vi "user_PW_dialog.vi"() -> (3 "result":bool)   [LabVIEW 2022 SP3]
uses:
  <vilib>/Utility/miscctls.llb/LVPointTypeDef.ctl
panel:
  in  "退出":bool
  in  "登录":bool
  out "登陆结果":string
  in  "密码":string
  in  "用户名":string
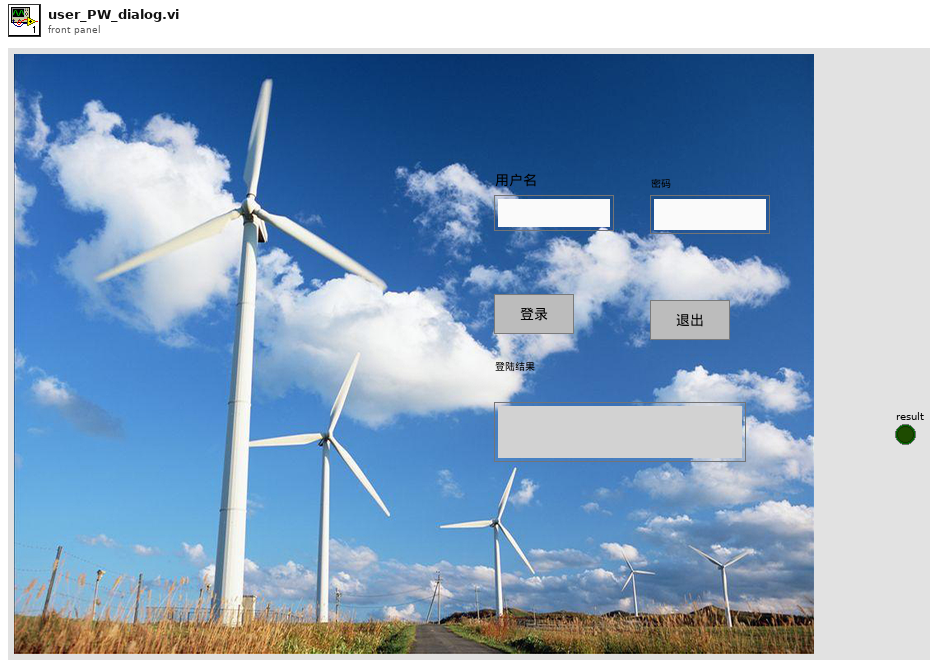
[diagram p1: front panel]
types:
  T1 = typedef "LVPointTypeDef.ctl" = cluster{"Horizontal":i16, "Vertical":i16}
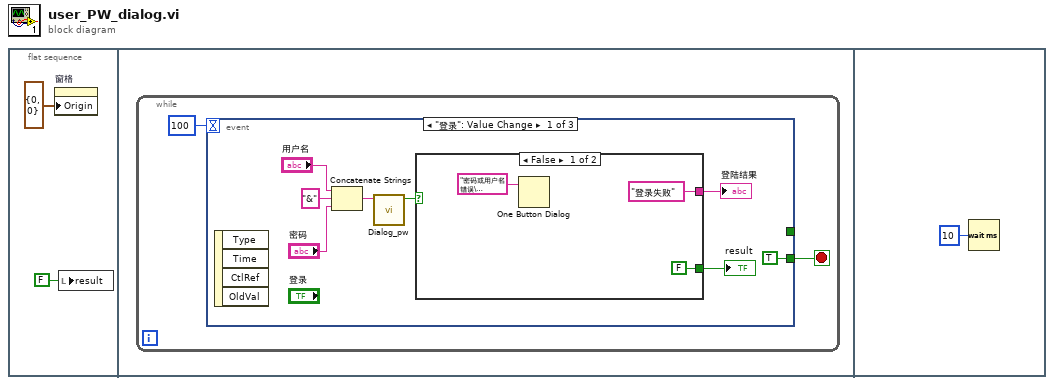
[diagram p0: block diagram]
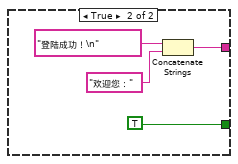
[diagram p2: hidden frame]
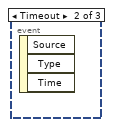
[diagram p3: hidden frame]
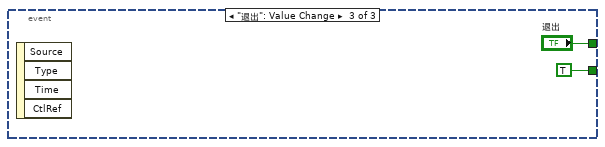
[diagram p4: hidden frame]
diagram:
  n1 = flat-sequence {
    frame #0 {
      n2 = property on="窗格" class="Pane"("Origin"=T1 {"Horizontal"=0, "Vertical"=0}) -> ()  [unwired: 2 in, 2 out]
      n3 = local write "result"(FALSE ("result")) -> ()
    }
    frame #1 {
      n4 = while {
        stop <- w3 stop-if-true
        n5 = event shown="[0] \"登录\": Value Change" {
          selector: _ -> [_ _ _]
          dyn-events: _ -> [_ _ _]
          timeout: 100 -> [_ _ _]
          tunnel: [_ _ "退出"] -> _
          tunnel: [TRUE _ TRUE] -> w3
          event "登录": Value Change {
            n6 = event-data() -> ()  [unwired: 5 out]
            n7 = Concatenate Strings("用户名", "&" ("string"), "密码") -> (w8:string)
            n8 = call "Dialog_pw.vi"("String"=w8) -> ("x >= 0?"=w7:bool)  [unwired: 10 in]
            n9 = case shown="False" w7 {
              tunnel: ["登录失败" w17] -> w10
              tunnel: [FALSE TRUE] -> w6
              frame False {
                n10 = One Button Dialog(message="密码或用户名错误\n请重新输入") -> ()  [unwired: 2 out]
              }
              frame True {
                n11 = Concatenate Strings("登陆成功！\n", "欢迎您：") -> (w17:string)
              }
            }
            "登陆结果" <- w10
            "result" <- w6
          }
          event Timeout {
            n12 = event-data() -> ()  [unwired: 4 out]
          }
          event "退出": Value Change {
            n13 = event-data() -> ()  [unwired: 5 out]
          }
        }
      }
    }
    frame #2 {
      n14 = Wait (ms)(milliseconds to wait=u32 10) -> ()  [unwired: 1 out]
    }
  }
